vi "DE_Eval Objective and Constraint.vi"(5 "function data":variant, 6 "stopping state in":T1={"max iterations"=50, "max function calls"=-1, "max time (sec)"=-1.0, "cur function calls"=0, "init tick count"=0}, 7 "objective and constraint function":refnum<vi>, 8 "error in (no error)":errorcluster, 11 "State In":T2) -> (0 "error out":errorcluster, 3 "State Out":T2, 4 "stopping state out":T1={"max iterations"=50, "max function calls"=-1, "max time (sec)"=-1.0, "cur function calls"=0, "init tick count"=0})   [LabVIEW 2017, in "NI_AAL_GlobalOptimization.lvlib"]
uses:
  <vilib>/gmath/NI_AAL_GlobalOptimization.lvlib
  <vilib>/gmath/GlobalOptimization.llb/DE_State.ctl
  <vilib>/gmath/GlobalOptimization.llb/DE_Population.ctl
  <vilib>/gmath/GlobalOptimization.llb/DE_Stopping State.ctl
  <vilib>/gmath/NumericalOptimization/cno_output select.ctl
  <vilib>/gmath/NI_Gmath.lvlib
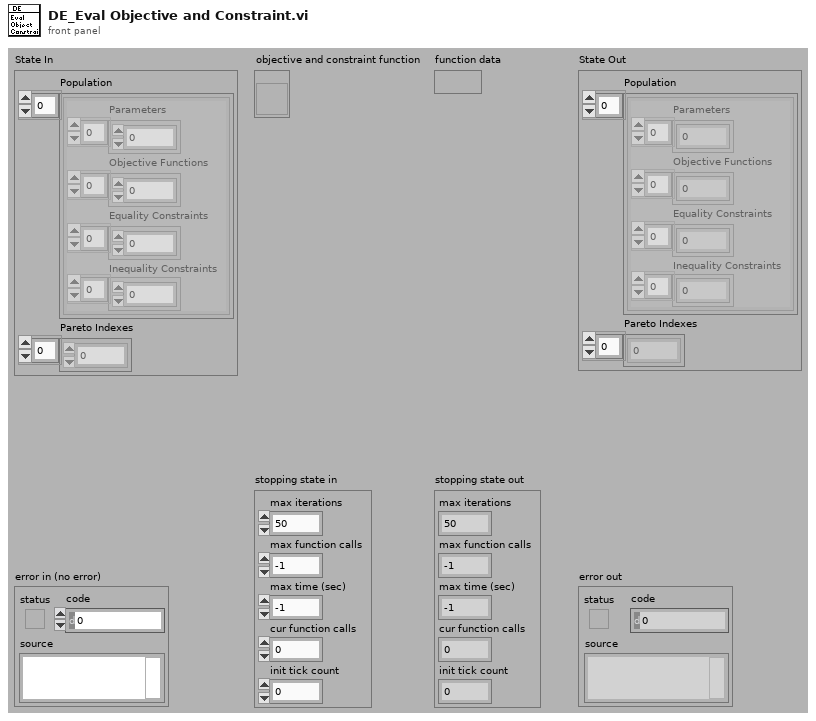
[diagram p1: front panel]
types:
  T1 = typedef "NI_AAL_GlobalOptimization.lvlib/DE_Stopping State.ctl" = cluster{"max iterations":i32, "max function calls":i32, "max time (sec)":dbl, "cur function calls":i32, "init tick count":u32}
  T2 = typedef "NI_AAL_GlobalOptimization.lvlib/DE_State.ctl" = cluster{"Population":T3[], "Pareto Indexes":i32[]}
  T3 = typedef "NI_AAL_GlobalOptimization.lvlib/DE_Population.ctl" = cluster{"Parameters":dbl[], "Objective Functions":dbl[], "Equality Constraints":dbl[], "Inequality Constraints":dbl[]}
  T4 = typedef "NI_Gmath.lvlib/cno_output select.ctl" = cluster{"objective function":bool, "equality constraint":bool, "inequality constraint":bool}
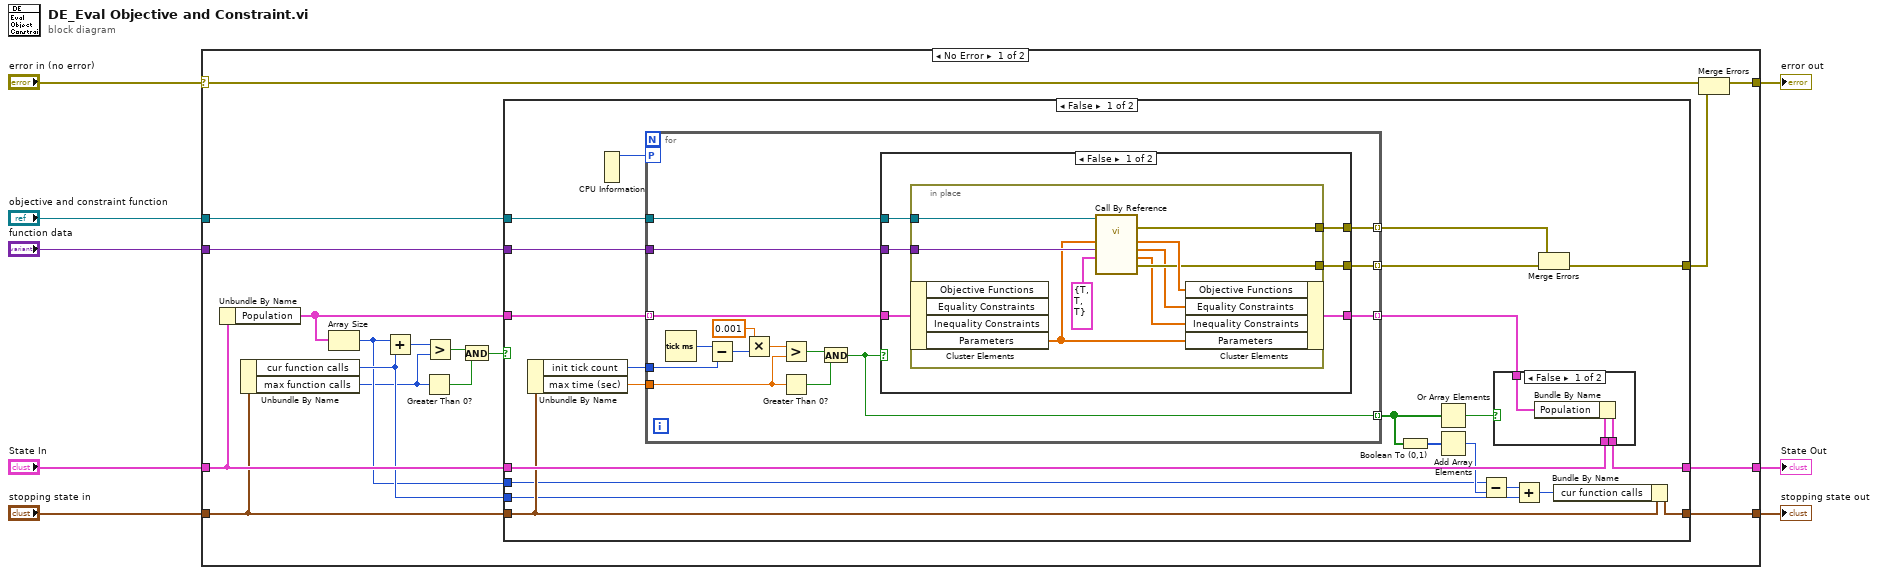
[diagram p0: block diagram]
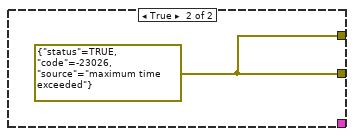
[diagram p3: hidden frame]
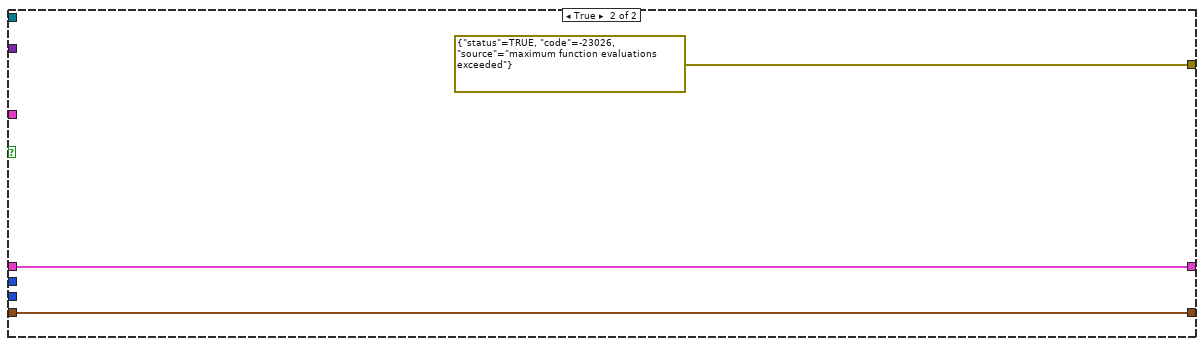
[diagram p4: hidden frame]
diagram:
  n1 = case shown="No Error" "error in (no error)" {
    selector: "error in (no error)" -> [w14 w87]
    tunnel: "function data" -> [w25 _]
    tunnel: "State In" -> [w24 w88]
    tunnel: [w23 w88] -> w6
    tunnel: "objective and constraint function" -> [w22 _]
    tunnel: [w15 w87] -> w3
    tunnel: "stopping state in" -> [w20 w86]
    tunnel: [w18 w86] -> w1
    frame No Error {
      n2 = Unbundle By Name(w24) -> ("Population"=w21:T3[])
      n3 = Unbundle By Name(w20) -> ("cur function calls"=w17:i32, "max function calls"=w12:i32)
      n4 = Array Size(array=w21) -> (size(s)=w13:i32)
      n5 = Add(x=w13, y=w17) -> (x+y=w19:i32)
      n6 = Greater Than 0?(x=w12) -> (x > 0?=w10:bool)
      n7 = Greater?(x=w19, y=w12) -> (0:w11:bool)
      n8 = And(x=w11, y=w10) -> (x .and. y?=w9:bool)
      n9 = case shown="False" w9 {
        tunnel: w25 -> [w46 _]
        tunnel: w24 -> [w45 w84]
        tunnel: [w44 w84] -> w23
        tunnel: [w42 errorcluster {"status"=TRUE, "code"=-23026, "source"="maximum function evaluations exceeded"} ("error out")] -> w16
        tunnel: w22 -> [w41 _]
        tunnel: w21 -> [w37 _]
        tunnel: w20 -> [w36 w85]
        tunnel: [w35 w85] -> w18
        tunnel: w17 -> [w34 _]
        tunnel: w13 -> [w28 _]
        frame False {
          n10 = Unbundle By Name(w36) -> ("init tick count"=w39:u32, "max time (sec)"=w38:dbl)
          n11 = CPU Information() -> (4:w47:i32)  [unwired: 3 out]
          n12 = for {
            tunnel: w46 -> [w66]
            tunnel: w37 -> [w65] mode=indexing
            workers-P: w47 -> [_]
            tunnel: [w64] -> w27 mode=indexing
            tunnel: [w63] -> w43 mode=indexing
            tunnel: w41 -> [w62]
            tunnel: [w61] -> w40 mode=indexing
            tunnel: w39 -> [w59]
            tunnel: w38 -> [w54]
            tunnel: [w52] -> w32 mode=indexing
            n13 = Tick Count (ms)() -> (millisecond timer value=w60:u32)
            n14 = Subtract(x=w60, y=w59) -> (x-y=w58:u32)
            n15 = Multiply(x=0.001 ("y"), y=w58) -> (x*y=w55:dbl)
            n16 = Greater?(x=w55, y=w54) -> (0:w53:bool)
            n17 = Greater Than 0?(x=w54) -> (x > 0?=w56:bool)
            n18 = And(x=w53, y=w56) -> (x .and. y?=w52:bool)
            n19 = case shown="False" w52 {
              tunnel: w66 -> [w72 _]
              tunnel: w65 -> [w71 _]
              tunnel: [w70 _] -> w64
              tunnel: [w69 w82] -> w63
              tunnel: w62 -> [w68 _]
              tunnel: [w67 w82] -> w61
              frame False {
                n20 = in-place {
                  in-place-border: w72 -> [w80]
                  in-place-border: [w79] -> w69
                  in-place-border: w68 -> [w75]
                  in-place-border: [w74] -> w67
                  n21 = in-place-cluster #1(w71) -> ("Parameters"=w78:dbl[])  [unwired: 3 out]
                  n22 = call-by-ref "?"(reference=w75, "output selector"=T4 {"objective function"=TRUE, "equality constraint"=TRUE, "inequality constraint"=TRUE}, "data"=w80, "X"=w78) -> (error out=w74:errorcluster, 0:"error out"=w79:errorcluster, "Inequality Constraints"=w77:dbl[], "Equality Constraints"=w76:dbl[], "Objective Functions"=w81:dbl[])  [unwired: 6 in, 1 out]
                  n23 = in-place-cluster #1("Objective Functions"=w81, "Equality Constraints"=w76, "Inequality Constraints"=w77, "Parameters"=w78) -> (w70:T3)
                }
              }
              frame True {
                w82 = errorcluster {"status"=TRUE, "code"=-23026, "source"="maximum time exceeded"} ("error out")
              }
            }
          }
          n24 = Boolean To (0,1)(Boolean=w32) -> (0, 1=w31:i16[])
          n25 = Or Array Elements(Boolean array=w32) -> (logical OR=w26:bool)
          n26 = Add Array Elements(numeric array=w31) -> (sum=w29:i16)
          n27 = Subtract(x=w28, y=w29) -> (x-y=w30:i32)
          n28 = case shown="False" w26 {
            tunnel: w45 -> [w50 w51]
            tunnel: [w49 w51] -> w44
            tunnel: w27 -> [w48 _]
            frame False {
              n29 = Bundle By Name(cluster=w50, "Population"=w48) -> (w49:T2)
            }
            frame True {
            }
          }
          n30 = Add(x=w30, y=w34) -> (x+y=w33:i32)
          n31 = Merge Errors(w40, w43) -> (w42:errorcluster)
          n32 = Bundle By Name(cluster=w36, "cur function calls"=w33) -> (w35:T1)
        }
        frame True {
        }
      }
      n33 = Merge Errors(w14, w16) -> (w15:errorcluster)
    }
    frame Error {
    }
  }
  "error out" <- w3
  "State Out" <- w6
  "stopping state out" <- w1
